vi "q1 minutes to hours and minutes.vi"() -> ()   [LabVIEW 2025]
panel:
  out "seconds":dbl
  out "hours":dbl
  in  "minutes":dbl
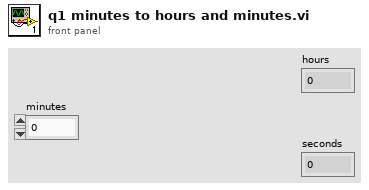
[diagram p1: front panel]
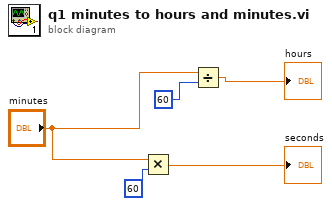
[diagram p0: block diagram]
diagram:
  n1 = Multiply(x="minutes", y=60) -> (x*y=→"seconds":dbl)
  n2 = Divide(x="minutes", y=60) -> (x/y=→"hours":dbl)
